vi "运维调试_总磷.vi"() -> ()   [LabVIEW 2016, in "总磷.lvlib"]
uses:
  <vilib>/Platform/TimedLoop/XDataNode/timing_clust.ctl
  <vilib>/Platform/TimedLoop/XDataNode/nitl_modes.ctl
  <vilib>/Platform/TimedLoop/XDataNode/wakeup.ctl
  <vilib>/Utility/miscctls.llb/LVPointTypeDef.ctl
  <vilib>/Platform/TimedLoop/XDataNode/XDataNode.xnode
  <vilib>/Platform/TimedLoop/XDataNode/XDNodeRunTimeDep.lvlib
panel:
  in  "数组":string[](array[string])
  in  "备用系数写入":bool
  in  "备用系数读取":bool
  in  "备用系数":T1
  in  "量程切换阈值写入":bool
  in  "量程切换阈值读取":bool
  in  "量程切换阈值":cluster{"阈值":dbl, "标液浓度":dbl}
  in  "参数下拉列表":enum16{"氨氮", "总磷"}(ring)=enum."总磷"
  in  "量程下拉列表":enum16{"低量程", "高量程"}(ring)
  in  "测量模式下拉列表":enum16{"水样测量", "空白核查", "标样核查", "盲样测试", "加标回收"}(ring)
  in  "公式":cluster{"X^2":dbl, "X":dbl, "b":dbl}
  in  "写公式":bool
  in  "读公式":bool
  in  "精度":dbl=4.0
  in  "样品5 F0":dbl
  in  "样品5 F1":dbl
  in  "样品4 F1":dbl
  in  "样品4 F0":dbl
  in  "样品3 F0":dbl
  in  "样品3 F1":dbl
  in  "样品2 F0":dbl
  in  "样品2 F1":dbl
  in  "样品1 F1":dbl
  in  "样品1 F0":dbl
  in  "method":u16(ring) items=["最小二乘", "最小绝对残差", "Bisquare"]
  in  "模型":enum32{"线性", "多项式"}(ring)
  out "r^2":dbl format="%.7g"
  out "拟合公式":string
  in  "样品2启用":bool
  in  "样品5启用":bool
  in  "样品4启用":bool
  in  "样品3启用":bool
  in  "样品1启用":bool
  in  "标液浓度5":dbl
  out "测量吸光度5":dbl
  in  "标液浓度4":dbl
  out "测量吸光度4":dbl
  in  "标液浓度3":dbl
  out "测量吸光度3":dbl
  in  "标液浓度2":dbl
  out "测量吸光度2":dbl
  out "测量吸光度1":dbl
  in  "标液浓度1":dbl
  out "XY图":cluster{"X Values":dbl[], "Y Values":dbl[]}[](graph)
  in  "返回":bool
  in  "调试":bool
  out "序列号":string="序列号"
  out "测量数据":T2(xcontrol)
  out "集成报警信息":string
  out "设置值":dbl
  out "定时启动":bool
  out "总磷总氮运行状态":T3(xcontrol)
  in  "停止":bool
  in  "手动启动":bool
  in  "单步测试":bool
  in  "总磷氨氮调试":u16[](xcontrol)
  out "F3":sgl format="%#.6f"
  out "F2":sgl format="%#.6f"
  out "F1":sgl format="%#.6f"
  out "F0":sgl format="%#.6f"
  out "多列列表框":i32(listbox)
  # "COM4"
  # "参数设置"
  # "标液浓度"
  # "F0"
  # "F1"
  # "吸光值显示"
  # "样品一"
  # "辅\n助\n计\n算\n区"
  # "样品二"
  # "样品三"
  # "样品四"
  # "样品五"
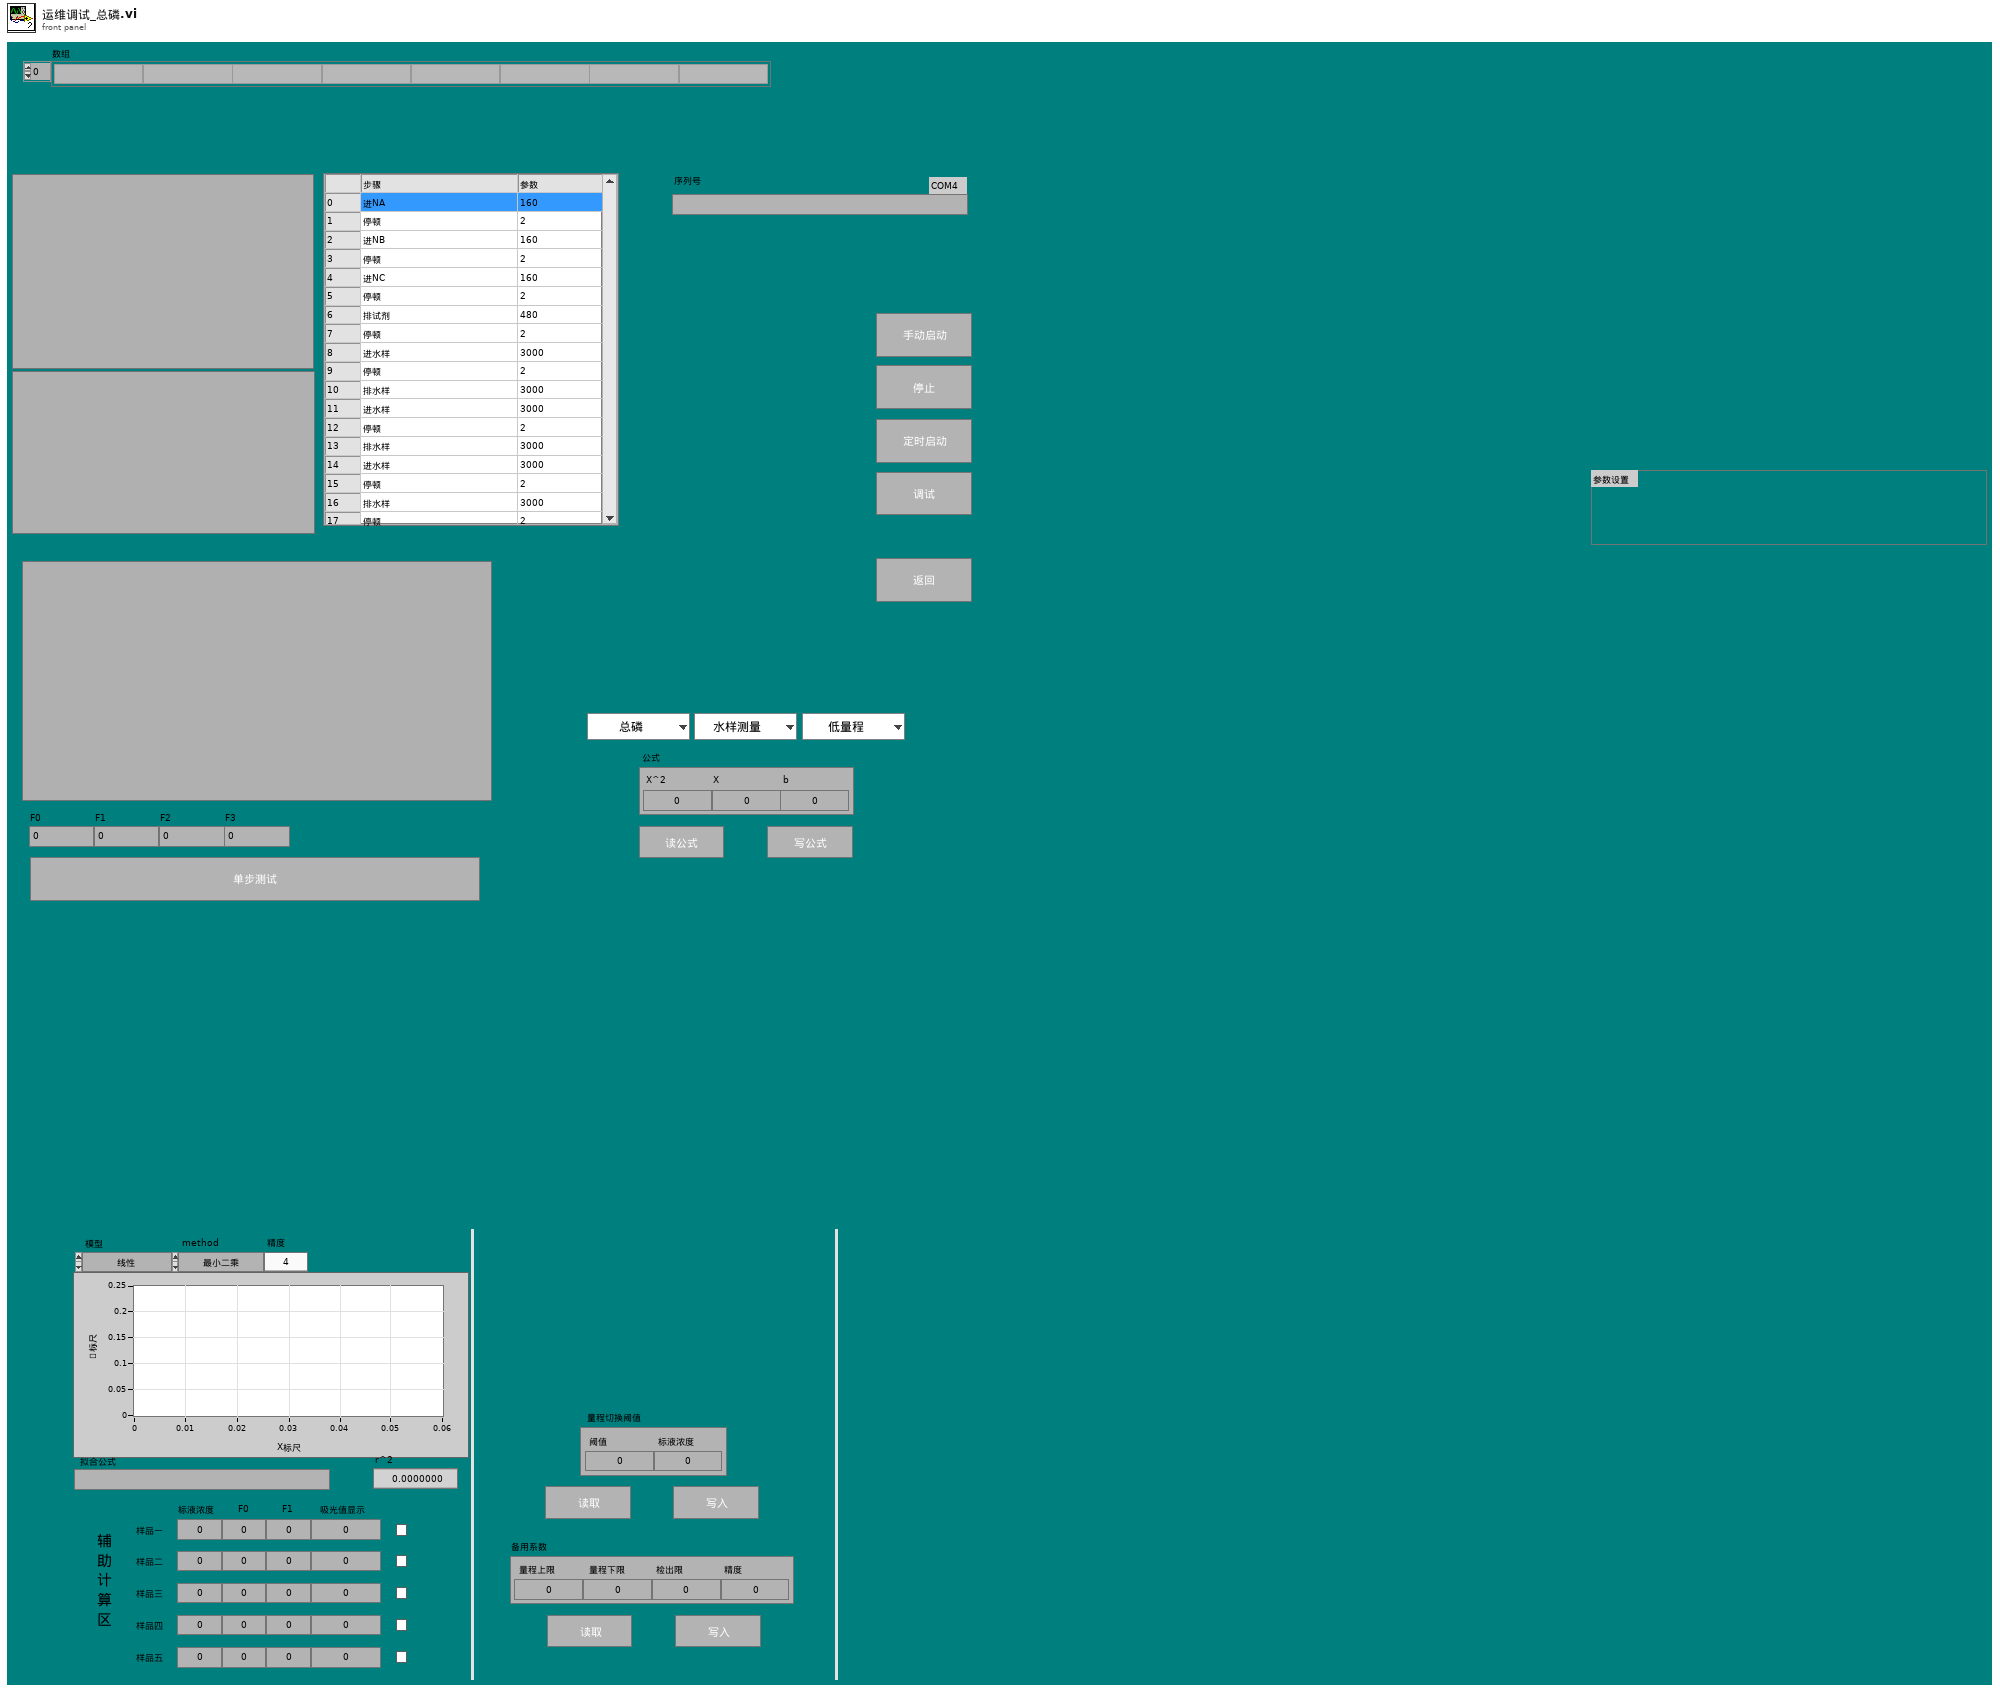
[diagram p1: front panel]
types:
  T1 = cluster{"量程上限":dbl, "量程下限":dbl, "检出限":dbl, "精度":dbl}
  T2 = cluster{"flowid":u16, "测量精度":u16, "测量数据区":cluster{"因子编码":u32, "单位":u16, "标样参考值":sgl, "水样数据时间":timestamp, "水样实测值":sgl, "水样数据标识":string, "标样数据时间":timestamp, "标样实测值":sgl, "标样数据标识":string, "空白数据时间":timestamp, "空白实测值":sgl, "空白数据标识":string, "零点核查数据时间":timestamp, "零点核查实测值":sgl, "零点核查数据标识":string, "跨度核查数据时间":timestamp, "跨度核查实测值":sgl, "跨度核查数据标识":string, "加标回收数据时间":timestamp, "加标回收实测值":sgl, "加标回收数据标识":string, "平行样数据时间":timestamp, "平行样实测值":sgl, "平行样数据标识":string}}
  T3 = cluster{"系统时间":timestamp, "工作状态":enum16{"空闲", "水样测试", "标样核查", "零点核查", "跨度核查", "空白测试", "平行样测试", "加标回收", "空白校准", "标样校准", "初始化（清洗）"}, "测量模式":enum16{"待机", "连续模式", "周期模式", "定点模式", "受控模式", "手动模式"}, "告警代码":enum16{"无告警", "缺试剂告警", "缺水样告警", "缺蒸馏水告警", "缺标液告警", "仪表漏液告警", "标定异常告警", "超量程告警", "加热异常", "低试剂预警", "超上限告警", "超下限告警", "仪表内部其他异常", "滴定异常告警", "电极异常告警", "量程切换告警", "参数设置告警", "PH电极电位异常", "电导率电极异常", "浊度光度异常", "溶解氧电极异常", "溶解氧光强异常", "温度异常告警", "PH异常告警", "溶解氧异常告警", "电导率异常告警", "浊度异常告警", "叶绿素异常告警", "藻密度异常告警", "蓝绿藻异常告警", "ORP异常告警", "氨氮异常告警", "清洁刷异常告警", "SD卡异常告警", "蓝牙异常告警", "Wifi异常告警", "流程异常告警"}, "故障代码":enum16{"无故障", "电机故障", "温度故障", "通讯故障", "滴定故障"}, "日志代码":u16, "软件版本":u16, "F0":sgl, "F1":sgl, "F2":sgl, "F3":sgl, "T":sgl, "H":sgl, "id":u16, "flowid":u16, "量程":u16}
  T4 = enum16{"待机", "启动氨氮", "氨氮测量中", "启动总磷", "总磷测量中", "延时"}
  T5 = typedef "LVPointTypeDef.ctl" = cluster{"Horizontal":i16, "Vertical":i16}
  T6 = cluster{"因子编码":u32, "单位":u16, "标样参考值":sgl, "水样数据时间":timestamp, "水样实测值":sgl, "水样数据标识":string, "标样数据时间":timestamp, "标样实测值":sgl, "标样数据标识":string, "空白数据时间":timestamp, "空白实测值":sgl, "空白数据标识":string, "零点核查数据时间":timestamp, "零点核查实测值":sgl, "零点核查数据标识":string, "跨度核查数据时间":timestamp, "跨度核查实测值":sgl, "跨度核查数据标识":string, "加标回收数据时间":timestamp, "加标回收实测值":sgl, "加标回收数据标识":string, "平行样数据时间":timestamp, "平行样实测值":sgl, "平行样数据标识":string}
  T7 = enum16{"空闲", "水样测试", "标样核查", "零点核查", "跨度核查", "空白测试", "平行样测试", "加标回收", "空白校准", "标样校准", "初始化（清洗）"}
  T8 = typedef "XDNodeRunTimeDep.lvlib/timing_clust.ctl" = cluster{"Expected End [f-1]":u64, "Actual End [f-1]":u64, "Finished Late? [f-1]":bool, "Expected End [i-1]":u64, "Actual End [i-1]":u64, "Finished Late? [i-1]":bool, "Expected Start [i]":u64, "Actual Start [i]":u64, "Expected Start [f]":u64, "Actual Start [f]":u64, "Source Name":string, "Structure Name":string, "Period":i64, "Deadline":i64, "Offset":i64, "Start":i64, "Priority":i32, "Timeout":i32, "Mode":T9, "Wakeup Reason":T10, "Error":errorcluster, "Source Type":string, "Secondary Source Type":string, "Global End Time":u64, "Global Start Time":u64, "Frame Duration":u64, "Iteration Duration":u64, "Assigned CPU":i32, "I/O Scan Engine Mode":u32}
  T9 = typedef "XDNodeRunTimeDep.lvlib/nitl_modes.ctl" = enum32{"No Change", "Process missed periods, maintain original phase", "Discard missed periods, maintain original phase", "Process missed periods, ignore original phase", "Discard missed periods, ignore original phase"}
  T10 = typedef "XDNodeRunTimeDep.lvlib/wakeup.ctl" = enum32{"Normal", "Aborted", "Asynchronous wakeup", "Timing source error", "Timed loop error", "Timeout"}
  T11 = cluster{"启动模式":enum16{"标液测量", "水样测量", "零液测量", "盲样测量", "加标回收"}, "启动参数":u16, "量程":enum16{"低量程", "高量程"}}
  T12 = cluster{"时间标识":timestamp, "设备":string, "日志信息":string, "流程参数":string}
  T13 = cluster{"时间标识":timestamp, "设备":string, "日志信息":string}
  T14 = enum16{"无告警", "缺试剂告警", "缺水样告警", "缺蒸馏水告警", "缺标液告警", "仪表漏液告警", "标定异常告警", "超量程告警", "加热异常", "低试剂预警", "超上限告警", "超下限告警", "仪表内部其他异常", "滴定异常告警", "电极异常告警", "量程切换告警", "参数设置告警", "PH电极电位异常", "电导率电极异常", "浊度光度异常", "溶解氧电极异常", "溶解氧光强异常", "温度异常告警", "PH异常告警", "溶解氧异常告警", "电导率异常告警", "浊度异常告警", "叶绿素异常告警", "藻密度异常告警", "蓝绿藻异常告警", "ORP异常告警", "氨氮异常告警", "清洁刷异常告警", "SD卡异常告警", "蓝牙异常告警", "Wifi异常告警", "流程异常告警"}
  T15 = typedef "LVRowAndColumnUnsignedTypeDef.ctl" = cluster{"Row":u32, "Column":u32}
  T16 = cluster{"站号":u16, "量程切换":enum32{"H", "L", "AUTO"}, "控制命令":enum16{"启动测量", "标样核查", "零点核查", "跨度核查", "空白测试", "平行样测试", "加标回收", "空白校准", "标样校准", "初始化（清洗）", "停止测试", "仪器重启", "校时", "模式设置", "测量间隔设置", "盲样测试"}, "模式设置":enum16{"待机", "连续模式", "周期模式", "定点模式", "受控模式", "手动模式"}, "测量间隔":u16}
  T17 = cluster{"站号":u16, "量程切换":enum32{"H", "L", "AUTO"}, "控制命令":enum16{"启动测量", "标样核查", "零点核查", "跨度核查", "空白测试", "平行样测试", "加标回收", "空白校准", "标样校准", "初始化（清洗）", "停止测试", "仪器重启", "校时", "模式设置", "测量间隔设置"}, "模式设置":enum16{"待机", "连续模式", "周期模式", "定点模式", "受控模式", "手动模式"}, "测量间隔":u16}
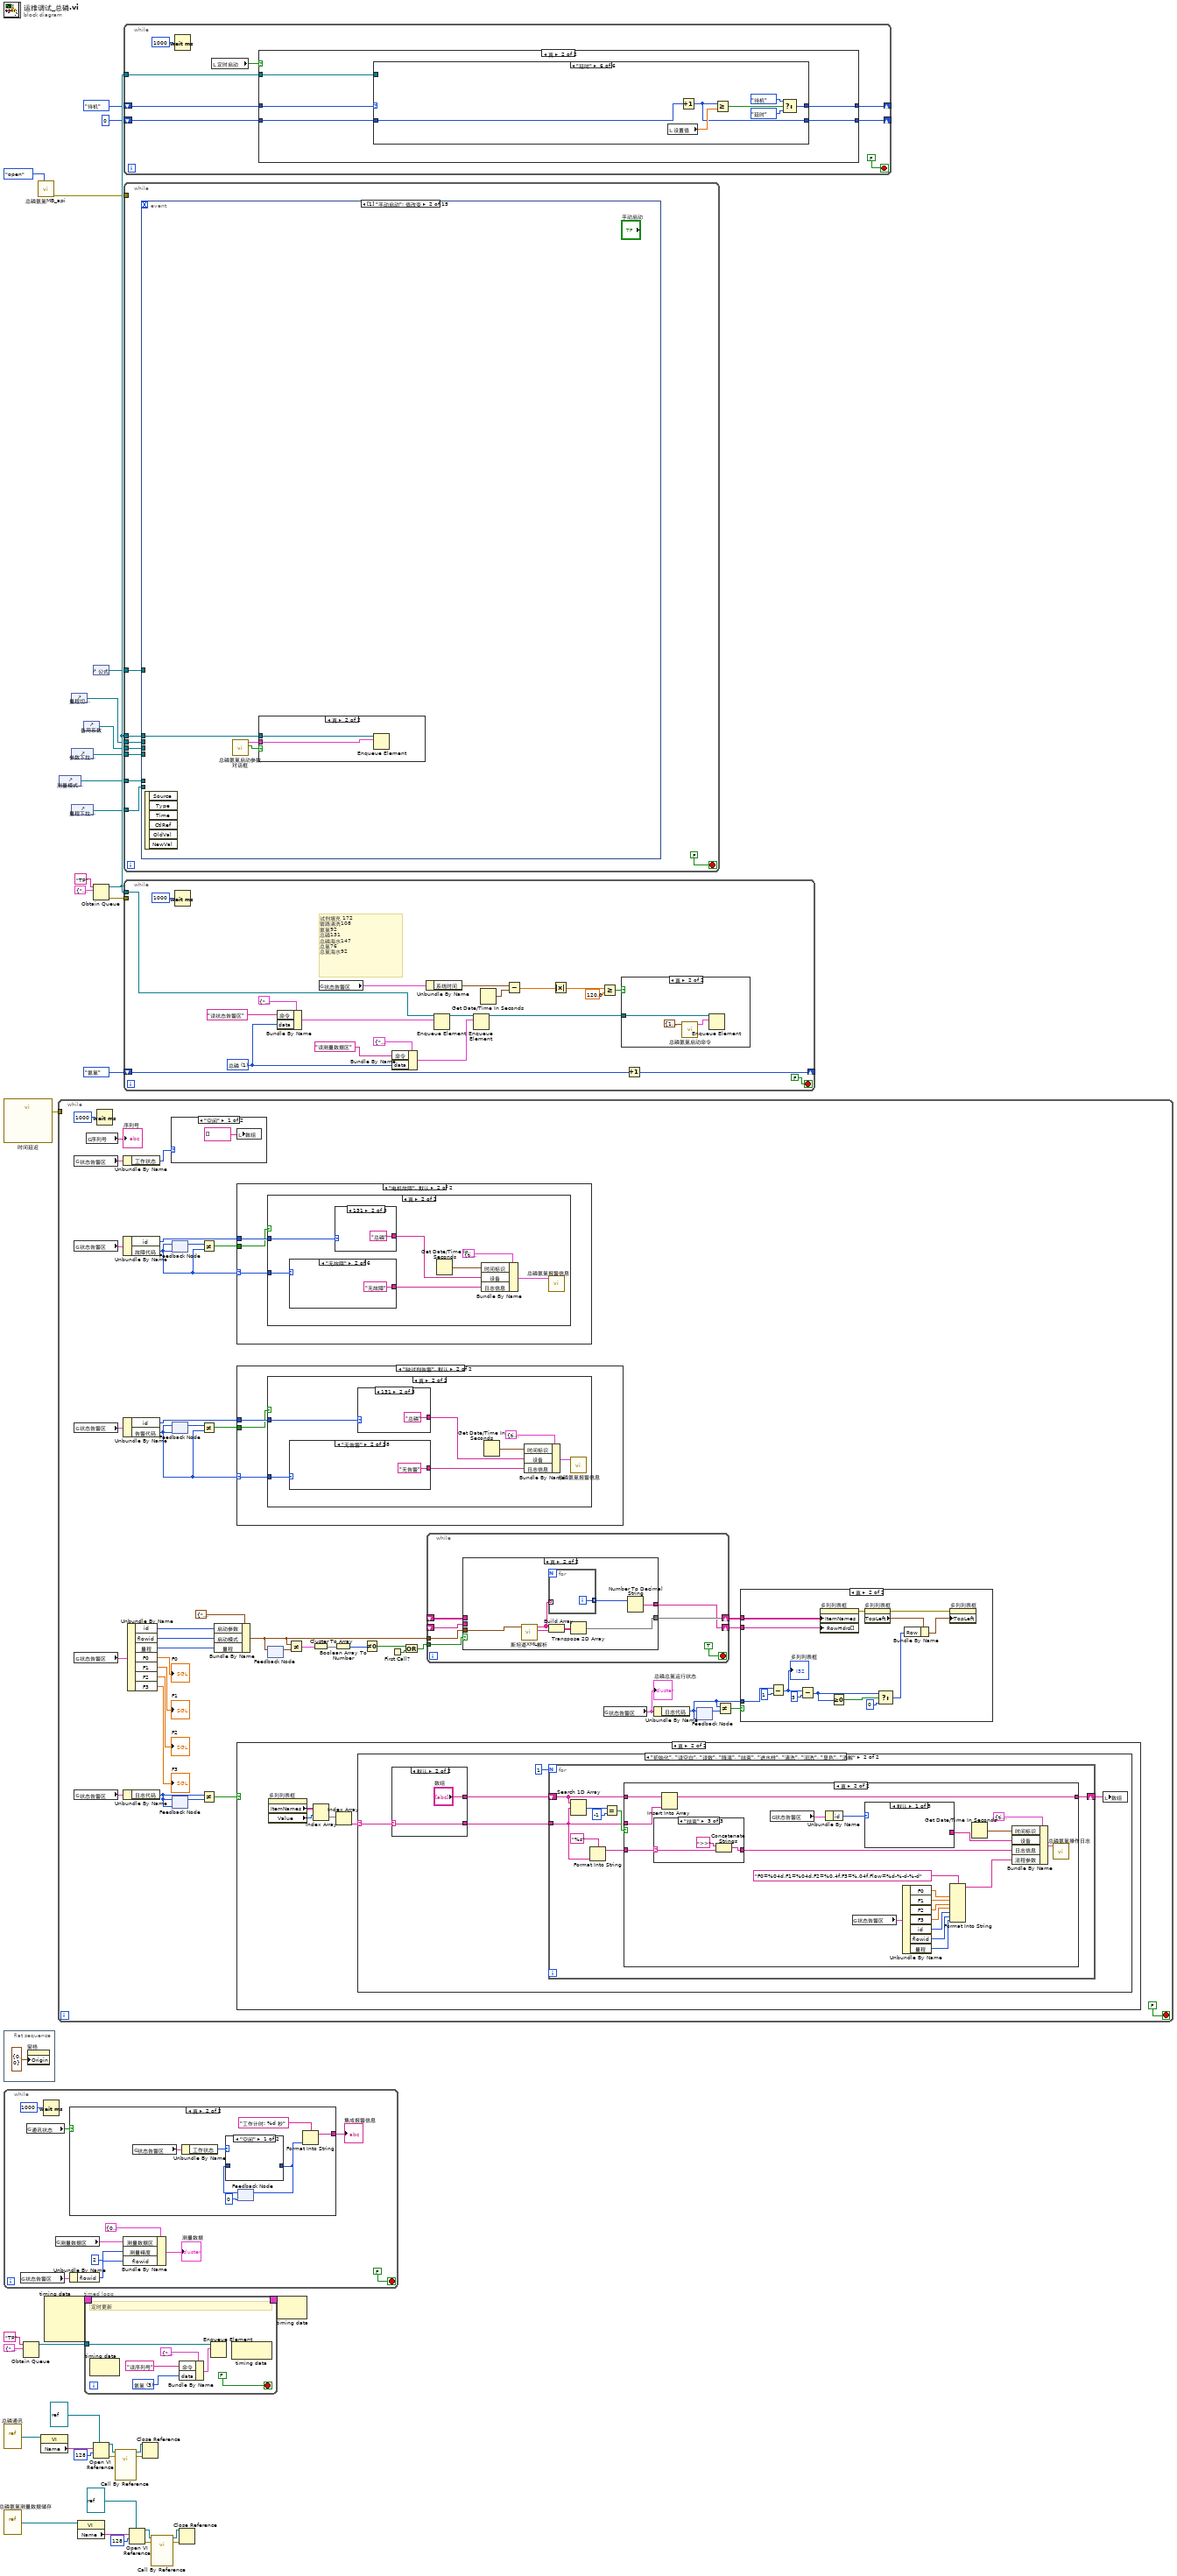
[diagram p0: block diagram]
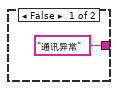
[diagram p2: hidden frame]
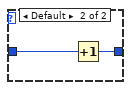
[diagram p3: hidden frame]
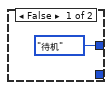
[diagram p4: hidden frame]
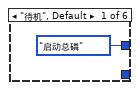
[diagram p5: hidden frame]
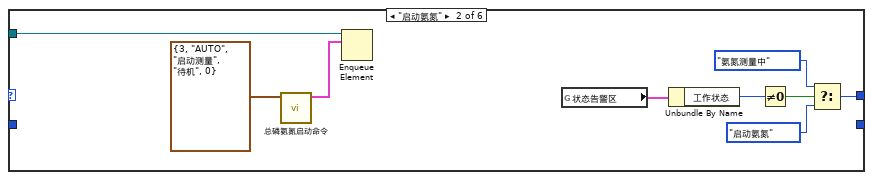
[diagram p6: hidden frame]
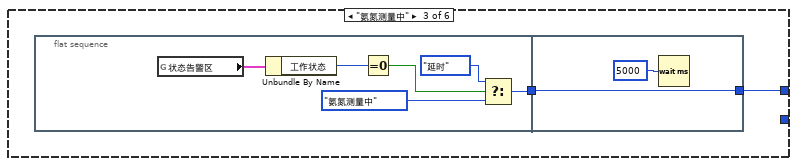
[diagram p7: hidden frame]
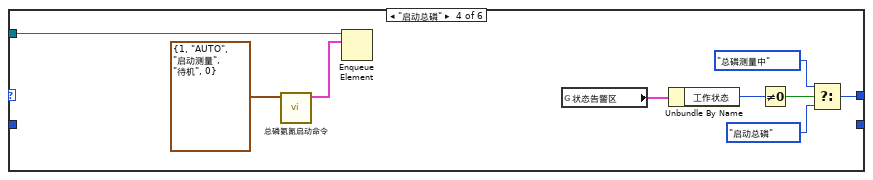
[diagram p8: hidden frame]
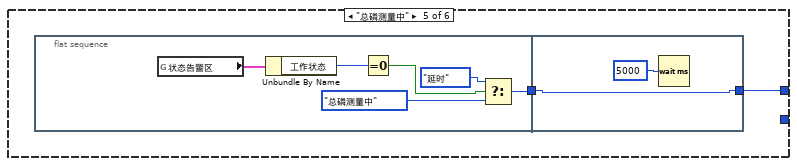
[diagram p9: hidden frame]
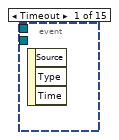
[diagram p10: hidden frame]
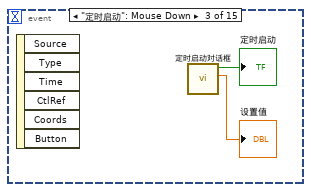
[diagram p12: hidden frame]
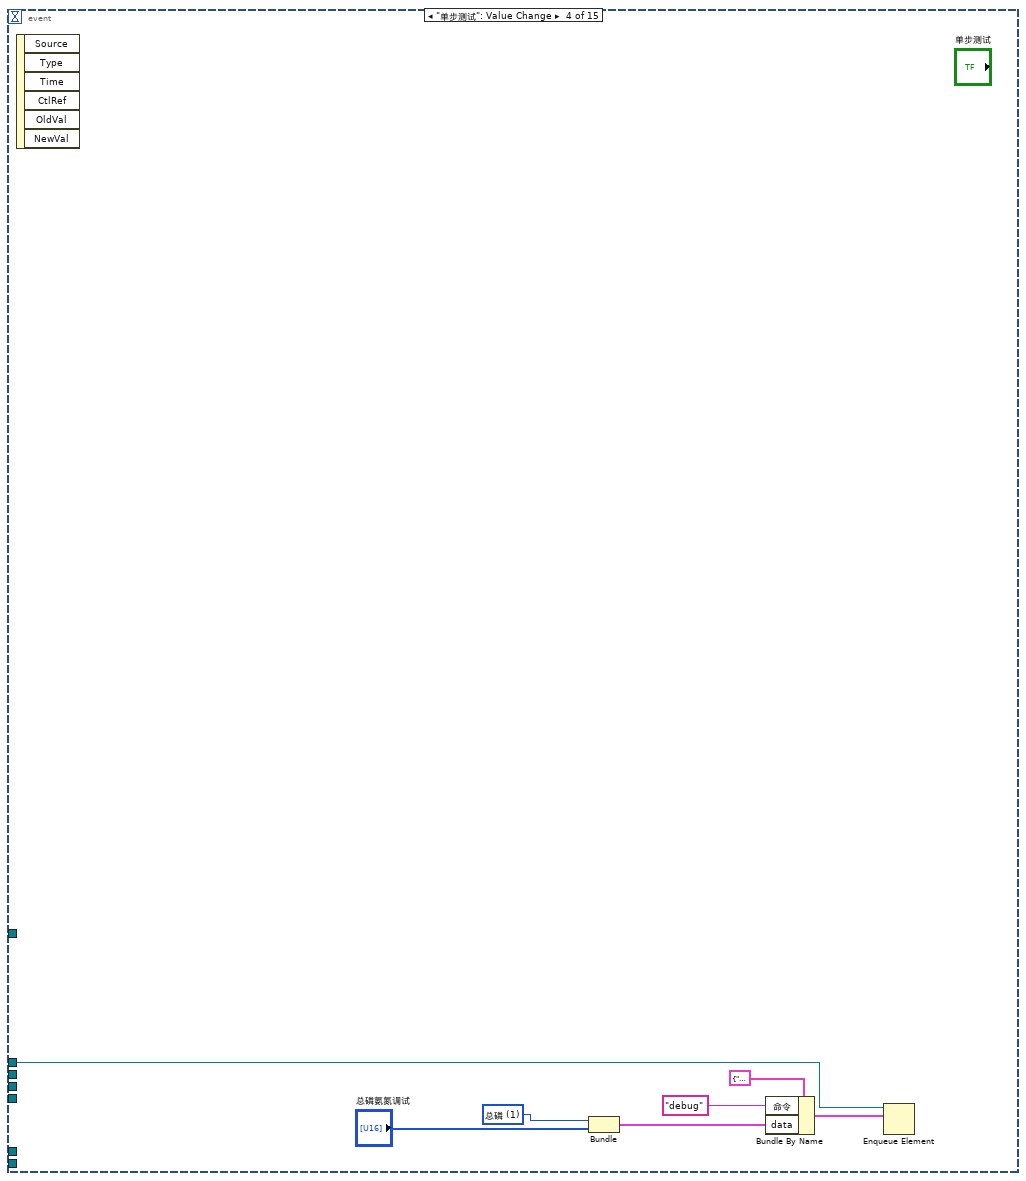
[diagram p13: hidden frame]
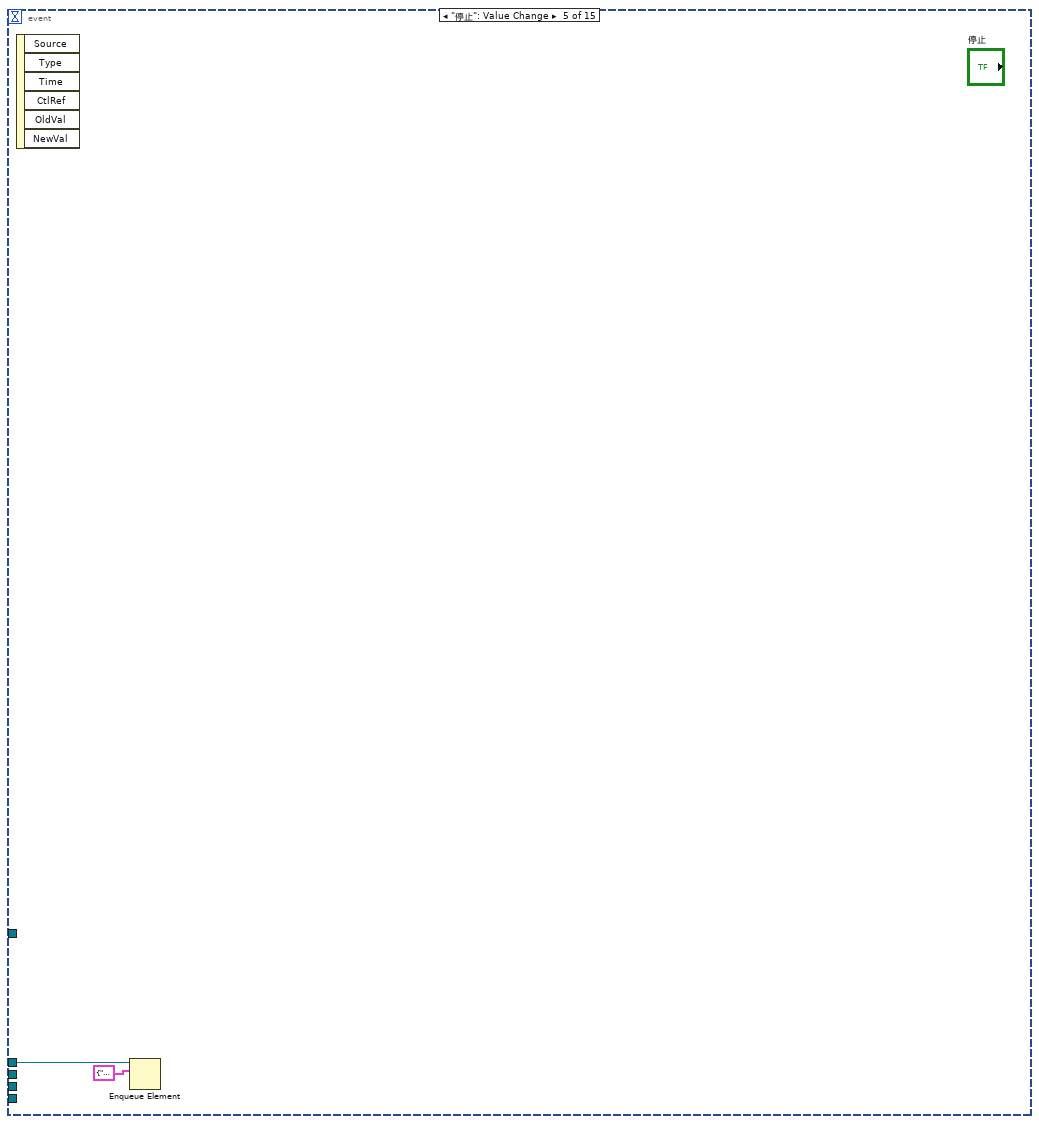
[diagram p14: hidden frame]
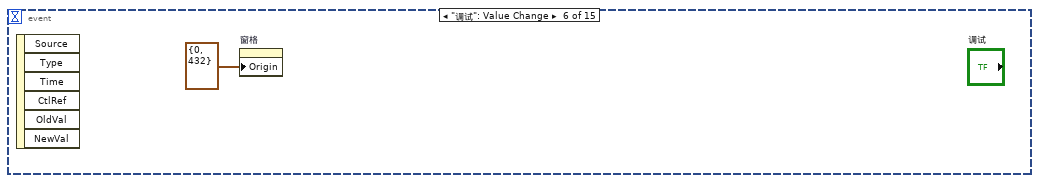
[diagram p15: hidden frame]
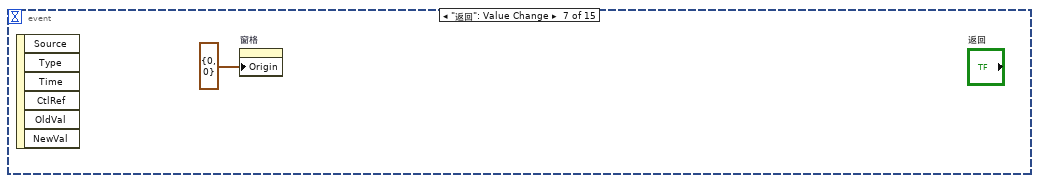
[diagram p16: hidden frame]
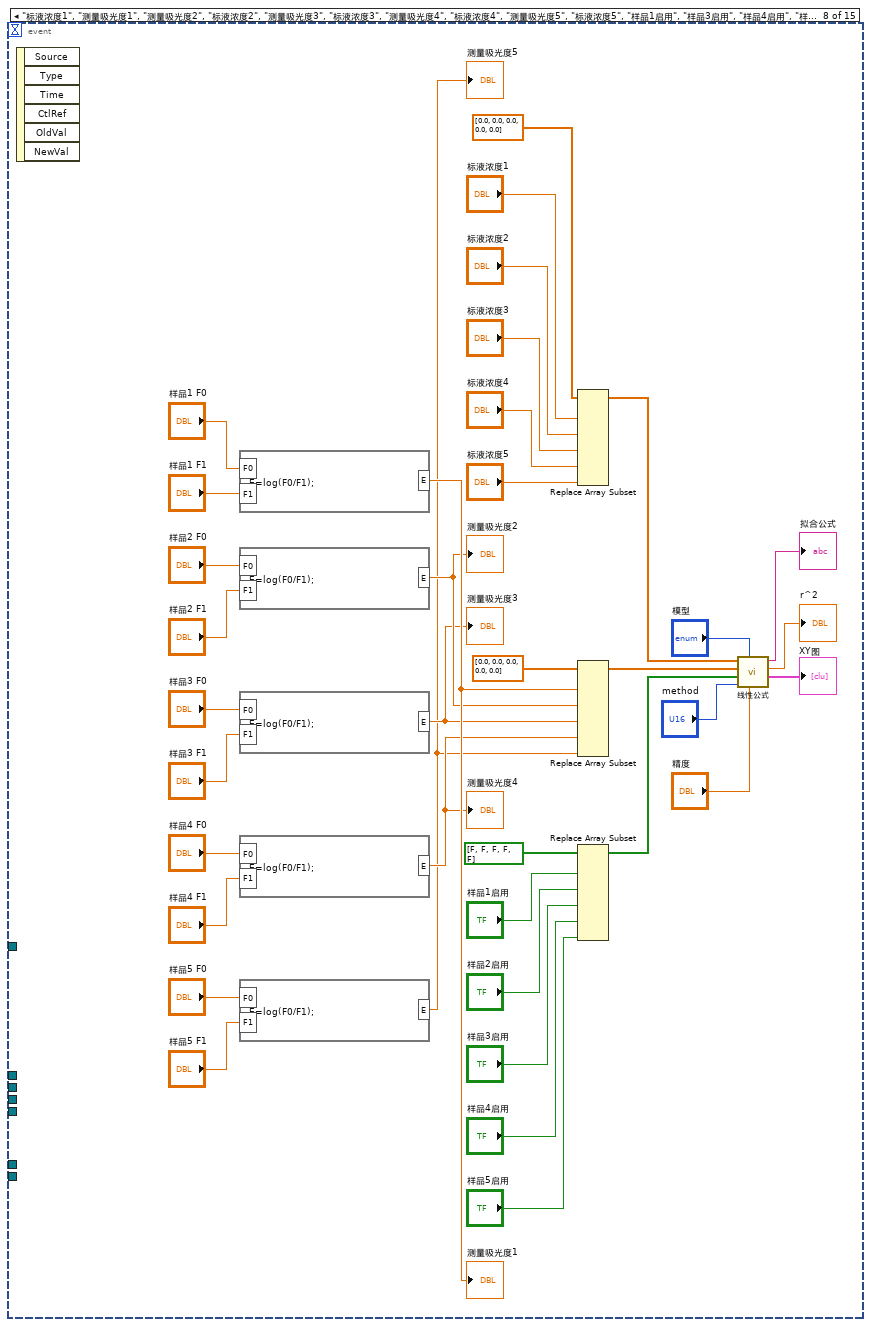
[diagram p17: hidden frame]
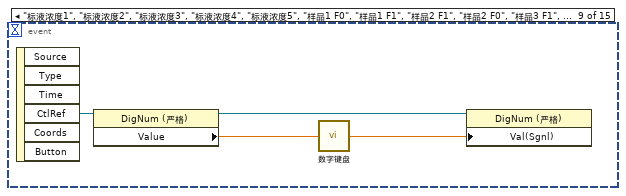
[diagram p18: hidden frame]
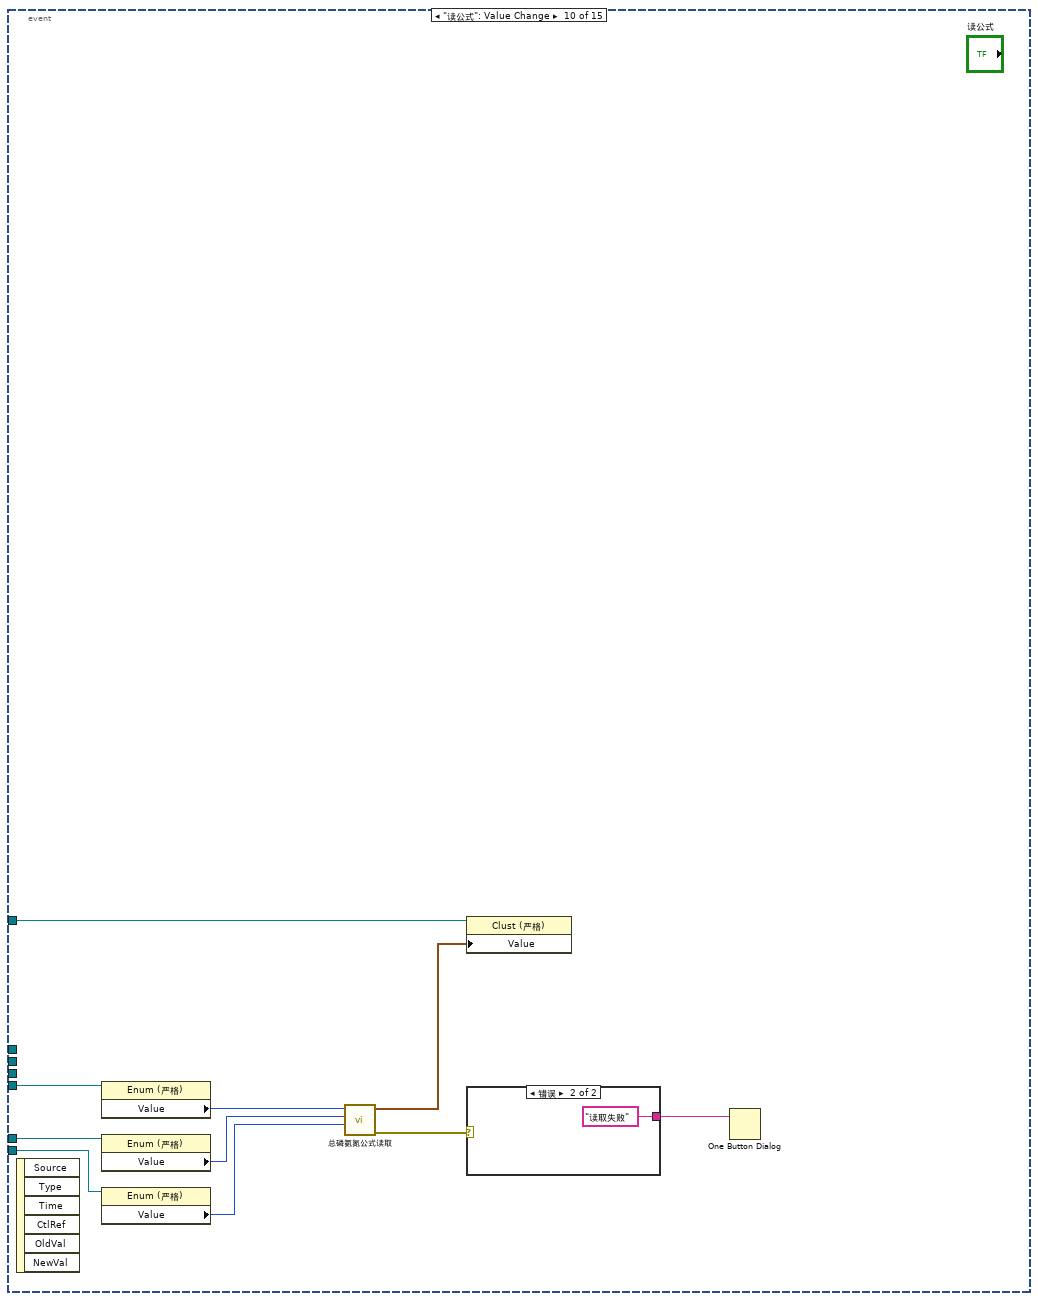
[diagram p19: hidden frame]
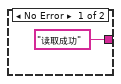
[diagram p20: hidden frame]
diagram:
  n1 = call "时间延迟"() -> ("error out"=w8:errorcluster)  [unwired: 11 in]
  n2 = flat-sequence {
    frame #0 {
      n3 = property on="窗格" class="Pane"("Origin"=T5 {"Horizontal"=0, "Vertical"=0} ("原点")) -> ()  [unwired: 2 in, 2 out]
    }
  }
  n4 = while {
    stop <- FALSE stop-if-true
    n5 = global read "VAR总磷氨氮全局变量.vi" "状态告警区"() -> (w43:T3)
    n6 = global read "VAR总磷氨氮全局变量.vi" "通讯状态"() -> (w45:bool)
    n7 = Wait (ms)(milliseconds to wait=u32 1000 ("等待时间（毫秒）")) -> ()  [unwired: 1 out]
    n8 = global read "VAR总磷氨氮全局变量.vi" "测量数据区"() -> (w46:T6)
    n9 = case shown="真" w45 {
      tunnel: ["通讯异常" ("集成报警信息") w50] -> w44
      frame False {
      }
      frame True {
        n10 = global read "VAR总磷氨氮全局变量.vi" "状态告警区"() -> (w56:T3)
        n11 = Unbundle By Name(w56) -> ("工作状态"=w55:T7)
        n12 = feedback #1(0) -> (w53:i32)
        n13 = case shown="\"空闲\"" w55 {
          tunnel: w53 -> [_ w58]
          tunnel: [_ w57] -> w51
          frame "空闲" {
          }
          frame Default {
            n14 = Increment(x=w58) -> (x+1=w57:i32)
          }
        }
        n15 = feedback-in #1(w51) -> ()
        n16 = Format Into String(format string="工作计时: %d 秒" ("格式字符串"), w51) -> (resulting string=w50:string)  [unwired: 2 in, 1 out]
      }
    }
    "集成报警信息" <- w44
    n17 = Unbundle By Name(w43) -> ("flowid"=w42:u16)
    n18 = Bundle By Name(cluster=T2 {"flowid"=0, "测量精度"=0, "测量数据区"={"因子编码"=0, "单位"=0, "标样参考值"=0.0, "水样数据时间"=timestamp(0 s since 1904-01-01), "水样实测值"=0.0, "水样数据标识"="", "标样数据时间"=timestamp(0 s since 1904-01-01), "标样实测值"=0.0, "标样数据标识"="", "空白数据时间"=timestamp(0 s since 1904-01-01), "空白实测值"=0.0, "空白数据标识"="", "零点核查数据时间"=timestamp(0 s since 1904-01-01), "零点核查实测值"=0.0, "零点核查数据标识"="", "跨度核查数据时间"=timestamp(0 s since 1904-01-01), "跨度核查实测值"=0.0, "跨度核查数据标识"="", "加标回收数据时间"=timestamp(0 s since 1904-01-01), "加标回收实测值"=0.0, "加标回收数据标识"="", "平行样数据时间"=timestamp(0 s since 1904-01-01), "平行样实测值"=0.0, "平行样数据标识"=""}} ("氨氮测量数据"), "测量数据区"=w46, "测量精度"=u16 2, "flowid"=w42) -> (→"测量数据":T2)
  }
  n19 = vi-ref "总磷通讯.vi"() -> (w31:refnum<vi>)
  n20 = vi-ref "总磷氨氮测量数据储存.vi"() -> (w23:refnum<vi>)
  n21 = Obtain Queue(name (unnamed)="TP" ("名称（未命名）"), element data type=cluster{"命令":string, "data":variant} {"命令"="", "data"=variant}) -> (queue out=w1:refnum<queue>)  [unwired: 3 in, 2 out]
  n22 = call "总磷氨氮MB_api.vi"("STEP"=enum16{"open", "read", "write", "close"}."open") -> ("error out"=w7:errorcluster)  [unwired: 8 in, 2 out]
  n23 = property class="VI"(reference=w31) -> ("Name"=w30:string)  [unwired: 1 in, 2 out]
  n24 = node-c288() -> (w5:T8)  [unwired: 4 in]
  n25 = while {
    tunnel: w8 -> [_]
    stop <- FALSE stop-if-true
    n26 = global read "VAR总磷氨氮全局变量.vi" "状态告警区"() -> (w64:T3)
    n27 = global read "VAR总磷氨氮全局变量.vi" "状态告警区"() -> (w70:T3)
    n28 = global read "VAR总磷氨氮全局变量.vi" "状态告警区"() -> (w75:T3)
    n29 = global read "VAR总磷氨氮全局变量.vi" "状态告警区"() -> (w87:T3)
    n30 = global read "VAR总磷氨氮全局变量.vi" "状态告警区"() -> (w61:T3)
    n31 = global read "VAR总磷氨氮全局变量.vi" "序列号"() -> (→"序列号":string)
    n32 = Wait (ms)(milliseconds to wait=u32 1000 ("等待时间（毫秒）")) -> ()  [unwired: 1 out]
    n33 = Unbundle By Name(w64) -> ("工作状态"=w63:T7)
    n34 = Unbundle By Name(w70) -> ("id"=w69:u16, "故障代码"=w66:enum16{"无故障", "电机故障", "温度故障", "通讯故障", "滴定故障"})
    n35 = Unbundle By Name(w75) -> ("id"=w74:u16, "告警代码"=w71:T14)
    n36 = Unbundle By Name(w61) -> ("日志代码"=w60:u16)
    n37 = Unbundle By Name(w87) -> ("id"=w84:u16, "flowid"=w86:u16, "量程"=w85:u16, "F0"=→"F0":sgl, "F1"=→"F1":sgl, "F2"=→"F2":sgl, "F3"=→"F3":sgl)
    n38 = case shown="\"空闲\"" w63 {
      frame "空闲" {
        n39 = local write "数组"(string[] [] ("数组")) -> ()
      }
      frame "水样测试", Default {
      }
    }
    n40 = feedback #2(w66) -> (w67:enum16{"无故障", "电机故障", "温度故障", "通讯故障", "滴定故障"})
    n41 = feedback-in #2(w66) -> ()
    n42 = feedback #3(w71) -> (w72:T14)
    n43 = feedback-in #3(w71) -> ()
    n44 = feedback #4(w60) -> (w62:u16)
    n45 = feedback-in #4(w60) -> ()
    n46 = Not Equal?(x=w67, y=w66) -> (x != y?=w68:bool)
    n47 = Not Equal?(x=w72, y=w71) -> (x != y?=w73:bool)
    n48 = Not Equal?(x=w60, y=w62) -> (x != y?=w59:bool)
    n49 = Bundle By Name(cluster=T11 {"启动模式"=enum."加标回收", "启动参数"=1, "量程"=enum."低量程"} ("参数簇"), "启动参数"=w84, "启动模式"=w86, "量程"=w85) -> (w77:T11)
    n50 = case shown="\"电机故障\", 默认" w66 {
      selector: w66 -> [_ w155]
      tunnel: w69 -> [_ w156]
      tunnel: w68 -> [_ w154]
      frame "无故障" {
      }
      frame "电机故障", Default {
        n51 = case shown="真" w154 {
          tunnel: w156 -> [_ w163]
          tunnel: w155 -> [_ w158]
          frame False {
          }
          frame True {
            n52 = case shown="\"无故障\"" w158 {
              selector: w158 -> [w165 _ _ _ _ _]
              tunnel: [w164 "无故障" "电机故障" "温度故障" "通讯故障" "滴定故障"] -> w157
              frame Default {
                n53 = Format Into String(format string="%d" ("格式字符串"), initial string="未知" ("工作状态"), w165) -> (resulting string=w164:string)  [unwired: 1 in, 1 out]
              }
              frame "无故障" {
              }
              frame "电机故障" {
              }
              frame "温度故障" {
              }
              frame "通讯故障" {
              }
              frame "滴定故障" {
              }
            }
            n54 = case shown="131" w163 {
              tunnel: [_ "总磷" ("table输入") "氨氮" ("table输入")] -> w159
              frame Default {
              }
              frame 131 {
              }
              frame 92 {
              }
            }
            n55 = Get Date/Time In Seconds() -> (seconds since 1Jan1904=w160:timestamp)
            n56 = Bundle By Name(cluster=T13 {"时间标识"=timestamp(0 s since 1904-01-01), "设备"="", "日志信息"=""} ("data in"), "时间标识"=w160, "设备"=w159, "日志信息"=w157) -> (w161:T13)
            n57 = call "总磷氨氮报警信息.vi"("data in"=w161) -> ()  [unwired: 11 in]
          }
        }
      }
    }
    n58 = case shown="\"缺试剂告警\", 默认" w71 {
      selector: w71 -> [_ w176]
      tunnel: w74 -> [_ w177]
      tunnel: w73 -> [_ w175]
      frame "无告警" {
      }
      frame "缺试剂告警", Default {
        n59 = case shown="真" w175 {
          tunnel: w177 -> [_ w184]
          tunnel: w176 -> [_ w178]
          frame False {
          }
          frame True {
            n60 = case shown="\"无告警\"" w178 {
              selector: w178 -> [w186 _ _ _ _ _ _ _ _ _ _ _ _ _ _ _ _ _ _ _ _ _ _ _ _ _ _ _ _ _ _ _ _ _ _ _ _ _]
              tunnel: [w185 "无告警" "缺试剂告警" "缺水样告警" "缺蒸馏水告警" "缺标液告警" "仪表漏液告警" "标定异常告警" "超量程告警" "加热异常" "低试剂预警" "超上限告警" "超下限告警" "仪表内部其他异常" "滴定异常告警" "电极异常告警" "量程切换告警" "参数设置告警" "PH电极电位异常" "电导率电极异常" "浊度光度异常" "溶解氧电极异常" "溶解氧光强异常" "温度异常告警" "PH异常告警" "溶解氧异常告警" "电导率异常告警" "浊度异常告警" "叶绿素异常告警" "藻密度异常告警" "蓝绿藻异常告警" "ORP异常告警" "氨氮异常告警" "清洁刷异常告警" "SD卡异常告警" "蓝牙异常告警" "WiFi异常告警" "流程异常告警"] -> w179
              frame Default {
                n61 = Format Into String(format string="%d" ("格式字符串"), initial string="未知" ("工作状态"), w186) -> (resulting string=w185:string)  [unwired: 1 in, 1 out]
              }
              frame "无告警" {
              }
              frame "缺试剂告警" {
              }
              frame "缺水样告警" {
              }
              frame "缺蒸馏水告警" {
              }
              frame "缺标液告警" {
              }
              frame "仪表漏液告警" {
              }
              frame "标定异常告警" {
              }
              frame "超量程告警" {
              }
              frame "加热异常" {
              }
              frame "低试剂预警" {
              }
              frame "超上限告警" {
              }
              frame "超下限告警" {
              }
              frame "仪表内部其他异常" {
              }
              frame "滴定异常告警" {
              }
              frame "电极异常告警" {
              }
              frame "量程切换告警" {
              }
              frame "参数设置告警" {
              }
              frame "PH电极电位异常" {
              }
              frame "电导率电极异常" {
              }
              frame "浊度光度异常" {
              }
              frame "溶解氧电极异常" {
              }
              frame "溶解氧光强异常" {
              }
              frame "温度异常告警" {
              }
              frame "PH异常告警" {
              }
              frame "溶解氧异常告警" {
              }
              frame "电导率异常告警" {
              }
              frame "浊度异常告警" {
              }
              frame "叶绿素异常告警" {
              }
              frame "藻密度异常告警" {
              }
              frame "蓝绿藻异常告警" {
              }
              frame "ORP异常告警" {
              }
              frame "氨氮异常告警" {
              }
              frame "清洁刷异常告警" {
              }
              frame "SD卡异常告警" {
              }
              frame "蓝牙异常告警" {
              }
              frame "Wifi异常告警" {
              }
              frame "流程异常告警" {
              }
            }
            n62 = case shown="131" w184 {
              tunnel: [_ "总磷" ("table输入") "氨氮" ("table输入")] -> w180
              frame Default {
              }
              frame 131 {
              }
              frame 92 {
              }
            }
            n63 = Get Date/Time In Seconds() -> (seconds since 1Jan1904=w181:timestamp)
            n64 = Bundle By Name(cluster=T13 {"时间标识"=timestamp(0 s since 1904-01-01), "设备"="", "日志信息"=""} ("data in"), "时间标识"=w181, "设备"=w180, "日志信息"=w179) -> (w182:T13)
            n65 = call "总磷氨氮报警信息.vi"("data in"=w182) -> ()  [unwired: 11 in]
          }
        }
      }
    }
    n66 = case shown="真" w59 {
      frame False {
      }
      frame True {
        n67 = property on="多列列表框" class="MCListbox (严格)"() -> ("ItemNames"=w104:string[][], "Value"=w105:i32)  [unwired: 2 in, 2 out]
        n68 = Index Array(array=w104, index (row)=w105) -> (element=w103:string[])  [unwired: 1 in]
        n69 = Index Array(array=w103) -> (element=w102:string)  [unwired: 1 in]
        n70 = case shown="\"初始化\", \"读空白\", \"读数\", \"降温\", \"结束\", \"进水样\", \"清洗\", \"润洗\", \"显色\", \"消解\"" w102 {
          selector: w102 -> [_ w108]
          frame Default {
          }
          frame "初始化", "读空白", "读数", "降温", "结束", "进水样", "清洗", "润洗", "显色", "消解" {
            n71 = case shown="默认" w108 {
              selector: w108 -> [w112 w114]
              tunnel: [w112 w114] -> w107
              tunnel: [string[] [] ("数组") "数组"] -> w106
              frame "读数" {
              }
              frame Default {
              }
            }
            n72 = for {
              N: 1 -> [_]
              tunnel: w107 -> [w116]
              shift-right: [w115] -> w109
              shift-left: w106 -> [w117]
              n73 = Search 1D Array(1D array=w117, element=w116) -> (index of element=w120:i32)  [unwired: 1 in]
              n74 = Format Into String(format string="%s" ("格式字符串"), w116) -> (resulting string=w121:string)  [unwired: 2 in, 1 out]
              n75 = Equal?(x=w120, y=-1) -> (x = y?=w118:bool)
              n76 = case shown="真" w118 {
                tunnel: w121 -> [_ w125]
                tunnel: w117 -> [w123 w129]
                tunnel: w116 -> [_ w128]
                tunnel: [w123 w127] -> w115
                frame False {
                }
                frame True {
                  n77 = case shown="\"结束\"" w125 {
                    selector: w125 -> [w145 w148 w151]
                    tunnel: [w145 w147 w150] -> w124
                    frame Default {
                    }
                    frame "初始化" {
                      n78 = Concatenate Strings("<<" ("字符串"), w148) -> (w147:string)
                    }
                    frame "结束" {
                      n79 = Concatenate Strings(">>" ("字符串"), w151) -> (w150:string)
                    }
                  }
                  n80 = Insert Into Array(array=w129, new element=w128) -> (w127:string[])  [unwired: 1 in]
                  n81 = global read "VAR总磷氨氮全局变量.vi" "状态告警区"() -> (w144:T3)
                  n82 = Unbundle By Name(w144) -> ("id"=w143:u16)
                  n83 = global read "VAR总磷氨氮全局变量.vi" "状态告警区"() -> (w139:T3)
                  n84 = case shown="默认" w143 {
                    tunnel: [_ "总磷" ("table输入") "氨氮" ("table输入")] -> w141
                    frame Default {
                    }
                    frame 131 {
                    }
                    frame 92 {
                    }
                  }
                  n85 = Unbundle By Name(w139) -> ("F0"=w136:sgl, "F1"=w135:sgl, "F2"=w134:sgl, "F3"=w133:sgl, "id"=w132:u16, "flowid"=w131:u16, "量程"=w130:u16)
                  n86 = Format Into String(format string="F0=%04d,F1=%04d,F2=%0.4f,F3=%.04f,Flow=%d-%-d-%-d" ("格式字符串"), w136, w135, w134, w133, w132, w131, w130) -> (resulting string=w137:string)  [unwired: 2 in, 1 out]
                  n87 = Get Date/Time In Seconds() -> (seconds since 1Jan1904=w140:timestamp)
                  n88 = Bundle By Name(cluster=T12 {"时间标识"=timestamp(0 s since 1904-01-01), "设备"="", "日志信息"="", "流程参数"=""} ("data in"), "时间标识"=w140, "设备"=w141, "日志信息"=w124, "流程参数"=w137) -> (w142:T12)
                  n89 = call "总磷氨氮操作日志.vi"("data in"=w142) -> ()  [unwired: 11 in]
                }
              }
            }
            n90 = local write "数组"(w109) -> ()
          }
        }
      }
    }
    n91 = feedback #5() -> (w93:T11)  [unwired: 1 in]
    n92 = feedback-in #5(w77) -> ()
    n93 = Not Equal?(x=w77, y=w93) -> (x != y?=w94:cluster{"启动模式":bool, "启动参数":bool, "量程":bool})
    n94 = Cluster To Array(cluster=w94) -> (array=w95:bool[])
    n95 = Boolean Array To Number(Boolean array=w95) -> (number=w96:u32)
    n96 = Not Equal To 0?(x=w96) -> (x != 0?=w89:bool)
    n97 = First Call?() -> (First Call?: T/F=w90:bool)
    n98 = Or(x=w89, y=w90) -> (x .or. y?=w88:bool)
    n99 = while {
      tunnel: w88 -> [w234]
      tunnel: w77 -> [w233]
      shift-right: [w232] -> w92
      shift-left: _ -> [w228]
      shift-right: [w231] -> w91
      shift-left: _ -> [w229]
      stop <- TRUE stop-if-true
      n100 = case shown="真" w234 {
        tunnel: [w236 w243] -> w231
        tunnel: [w235 w242] -> w232
        tunnel: w233 -> [_ w237]
        tunnel: w229 -> [w236 _]
        tunnel: w228 -> [w235 _]
        frame False {
        }
        frame True {
          n101 = call "斯坦道XML解析.vi"("参数簇"=w237) -> ("步骤时间"=w238:string[], "步骤名"=w240:string[])  [unwired: 9 in]
          n102 = for {
            tunnel: w240 -> [_] mode=indexing
            tunnel: [w244] -> w241 mode=indexing
            i -> [w244]
          }
          n103 = Build Array(w240, w238) -> (w239:string[][])
          n104 = Transpose 2D Array(2D array=w239) -> (transposed array=w242:string[][])
          n105 = Number To Decimal String(number=w241) -> (decimal integer string=w243:string[])  [unwired: 1 in]
        }
      }
    }
    n106 = global read "VAR总磷氨氮全局变量.vi" "状态告警区"() -> (w78:T3)
    "总磷总氮运行状态" <- w78
    n107 = Unbundle By Name(w78) -> ("日志代码"=w65:u16)
    n108 = feedback-in #6(w65) -> ()
    n109 = feedback #6(w65) -> (w98:u16)
    n110 = Not Equal?(x=w65, y=w98) -> (x != y?=w97:bool)
    n111 = case shown="真" w97 {
      tunnel: w65 -> [_ w247]
      tunnel: w92 -> [_ w254]
      tunnel: w91 -> [_ w253]
      frame False {
      }
      frame True {
        n112 = Subtract(x=w247, y=1) -> (x-y=w245:i32)
        "多列列表框" <- w245
        n113 = Subtract(x=w245, y=5) -> (x-y=w249:i32)
        n114 = property on="多列列表框" class="MCListbox (严格)"("ItemNames"=w254, "RowHdrs[]"=w253) -> (error out=w255:errorcluster)  [unwired: 2 in, 1 out]
        n115 = Greater Or Equal To 0?(x=w249) -> (x >= 0?=w248:bool)
        n116 = property on="多列列表框" class="MCListbox (严格)"(error in=w255) -> (error out=w256:errorcluster, "TopLeft"=w257:T15)  [unwired: 1 in, 1 out]
        n117 = Select(t=w249, s=w248, f=0) -> (s? t:f=w250:i32)
        n118 = Bundle By Name(cluster=w257, "Row"=w250) -> (w258:T15)
        n119 = property on="多列列表框" class="MCListbox (严格)"(error in=w256, "TopLeft"=w258) -> ()  [unwired: 1 in, 2 out]
      }
    }
  }
  n120 = control-ref of="测量模式下拉列表"() -> (w12:refnum<vi>)
  n121 = control-ref of="量程切换阈值"() -> (w10:refnum<vi>)
  n122 = control-ref of="参数下拉列表"() -> (w13:refnum<vi>)
  n123 = control-ref of="量程下拉列表"() -> (w14:refnum<vi>)
  n124 = property class="VI"(reference=w23) -> ("Name"=w16:string)  [unwired: 1 in, 2 out]
  n125 = control-ref of="备用系数"() -> (w9:refnum<vi>)
  n126 = timed-loop {
    timing: w5 -> [_]
    timing-out: [_] -> w4
    tunnel: w1 -> [w260]
    stop <- FALSE stop-if-true
    w261 = u16 3 items=["总磷"=1, "氨氮"=3] ("站号")
    # "定时更新"
    n127 = node-c288() -> ()  [unwired: 1 in, 1 out]
    n128 = Bundle By Name(cluster=cluster{"命令":string, "data":variant} {"命令"="", "data"=variant} ("元素"), "命令"="读序列号", "data"=w261) -> (w259:cluster{"命令":string, "data":variant})
    n129 = Enqueue Element(queue=w260, element=w259) -> ()  [unwired: 2 in, 3 out]
    n130 = node-c288() -> ()  [unwired: 1 in, 1 out]
  }
  n131 = control-ref of="公式"() -> (w11:refnum<vi>)
  n132 = Open VI Reference(type specifier VI Refnum (for type only)=refnum<vi> refnum, vi path=w30, options=128 ("选项")) -> (vi reference=w28:refnum<vi>, error out=w26:errorcluster)  [unwired: 3 in]
  n133 = Obtain Queue(name (unnamed)="TP" ("名称（未命名）"), element data type=cluster{"命令":string, "data":variant} {"命令"="", "data"=variant}) -> (queue out=w34:refnum<queue>, error out=w35:errorcluster)  [unwired: 3 in, 1 out]
  n134 = call-by-ref "?"(reference=w28, error in=w26) -> (reference out=w24:refnum<vi>, error out=w25:errorcluster)  [unwired: 12 in]
  n135 = while {
    tunnel: w34 -> [w269]
    shift-right: [w270] -> _
    shift-left: T4."待机" -> [w271]
    shift-right: [w267] -> _
    shift-left: u32 0 ("等待时间（毫秒）") -> [w268]
    stop <- FALSE stop-if-true
    n136 = Wait (ms)(milliseconds to wait=u32 1000 ("等待时间（毫秒）")) -> ()  [unwired: 1 out]
    n137 = local read "定时启动"() -> (w272:bool)
    n138 = case shown="真" w272 {
      tunnel: w271 -> [_ w280]
      tunnel: [T4."待机" w279] -> w270
      tunnel: w269 -> [_ w278]
      tunnel: w268 -> [_ w277]
      tunnel: [_ w276] -> w267
      frame False {
      }
      frame True {
        n139 = case shown="\"延时\"" w280 {
          tunnel: [T4."启动总磷" w285 w292 w303 w311 w323] -> w279
          tunnel: w278 -> [_ w290 _ w309 _ _]
          tunnel: w277 -> [_ _ _ _ _ w326]
          tunnel: [_ _ _ _ _ w322] -> w276
          frame "待机", Default {
          }
          frame "启动氨氮" {
            n140 = call "总磷氨氮启动命令.vi"("参数"=T16 {"站号"=3, "量程切换"=enum."AUTO", "控制命令"=enum."启动测量", "模式设置"=enum."待机", "测量间隔"=0}) -> ("启动命令"=w283:cluster{"命令":string, "data":variant})  [unwired: 10 in]
            n141 = Enqueue Element(queue=w290, element=w283) -> ()  [unwired: 2 in, 3 out]
            n142 = global read "VAR总磷氨氮全局变量.vi" "状态告警区"() -> (w289:T3)
            n143 = Unbundle By Name(w289) -> ("工作状态"=w288:T7)
            n144 = Not Equal To 0?(x=w288) -> (x != 0?=w287:bool)
            n145 = Select(t=T4."氨氮测量中", s=w287, f=T4."启动氨氮") -> (s? t:f=w285:T4)
          }
          frame "氨氮测量中" {
            n146 = flat-sequence {
              tunnel: [w296] -> w291
              tunnel: [w300] -> w292
              tunnel: w291 -> [w300]
              frame #0 {
                n147 = global read "VAR总磷氨氮全局变量.vi" "状态告警区"() -> (w297:T3)
                n148 = Unbundle By Name(w297) -> ("工作状态"=w298:T7)
                n149 = Equal To 0?(x=w298) -> (x = 0?=w293:bool)
                n150 = Select(t=T4."延时", s=w293, f=T4."氨氮测量中") -> (s? t:f=w296:T4)
              }
              frame #1 {
                n151 = Wait (ms)(milliseconds to wait=u32 5000 ("等待时间（毫秒）")) -> ()  [unwired: 1 out]
              }
            }
          }
          frame "启动总磷" {
            n152 = call "总磷氨氮启动命令.vi"("参数"=T16 {"站号"=1, "量程切换"=enum."AUTO", "控制命令"=enum."启动测量", "模式设置"=enum."待机", "测量间隔"=0}) -> ("启动命令"=w302:cluster{"命令":string, "data":variant})  [unwired: 10 in]
            n153 = Enqueue Element(queue=w309, element=w302) -> ()  [unwired: 2 in, 3 out]
            n154 = global read "VAR总磷氨氮全局变量.vi" "状态告警区"() -> (w304:T3)
            n155 = Unbundle By Name(w304) -> ("工作状态"=w305:T7)
            n156 = Not Equal To 0?(x=w305) -> (x != 0?=w306:bool)
            n157 = Select(t=T4."总磷测量中", s=w306, f=T4."启动总磷") -> (s? t:f=w303:T4)
          }
          frame "总磷测量中" {
            n158 = flat-sequence {
              tunnel: [w313] -> w310
              tunnel: [w319] -> w311
              tunnel: w310 -> [w319]
              frame #0 {
                n159 = global read "VAR总磷氨氮全局变量.vi" "状态告警区"() -> (w316:T3)
                n160 = Unbundle By Name(w316) -> ("工作状态"=w317:T7)
                n161 = Equal To 0?(x=w317) -> (x = 0?=w312:bool)
                n162 = Select(t=T4."延时", s=w312, f=T4."总磷测量中") -> (s? t:f=w313:T4)
              }
              frame #1 {
                n163 = Wait (ms)(milliseconds to wait=u32 5000 ("等待时间（毫秒）")) -> ()  [unwired: 1 out]
              }
            }
          }
          frame "延时" {
            n164 = local read "设置值"() -> (w325:dbl)
            n165 = Increment(x=w326) -> (x+1=w322:u32)
            n166 = Greater Or Equal?(x=w322, y=w325) -> (x >= y?=w324:bool)
            n167 = Select(t=T4."待机", s=w324, f=T4."延时") -> (s? t:f=w323:T4)
          }
        }
      }
    }
  }
  n168 = while {
    tunnel: w34 -> [w333]
    tunnel: w14 -> [w332]
    tunnel: w13 -> [w331]
    tunnel: w12 -> [w330]
    tunnel: w11 -> [w329]
    tunnel: w10 -> [w328]
    tunnel: w9 -> [w327]
    tunnel: w7 -> [_]
    stop <- FALSE stop-if-true
    n169 = event shown="[1] \"手动启动\": 值改变" {
      selector: _ -> [_ _ _ _ _ _ _ _ _ _ _ _ _ _ _]
      dyn-events: _ -> [_ _ _ _ _ _ _ _ _ _ _ _ _ _ _]
      timeout: _ -> [_ _ _ _ _ _ _ _ _ _ _ _ _ _ _]
      tunnel: w333 -> [_ w337 _ w348 w350 _ _ _ _ _ _ _ _ _ _]
      tunnel: w332 -> [_ _ _ _ _ _ _ _ _ w403 _ w423 w432 _ _]
      tunnel: w331 -> [_ _ _ _ _ _ _ _ _ w401 _ w421 w434 w442 w449]
      tunnel: w330 -> [_ _ _ _ _ _ _ _ _ w402 _ w422 w433 _ _]
      tunnel: w329 -> [_ _ _ _ _ _ _ _ _ w397 _ _ _ _ _]
      tunnel: w328 -> [_ _ _ _ _ _ _ _ _ _ _ w417 _ _ _]
      tunnel: w327 -> [_ _ _ _ _ _ _ _ _ _ _ _ _ w440 _]
      event Timeout {
        n170 = event-data() -> ()  [unwired: 1 in, 3 out]
      }
      event "手动启动": Value Change {
        n171 = event-data() -> ()  [unwired: 1 in, 6 out]
        n172 = call "总磷氨氮启动参数对话框.vi"() -> ("确认"=w335:bool, "元素"=w336:cluster{"命令":string, "data":variant})  [unwired: 10 in]
        n173 = case shown="真" w335 {
          tunnel: w337 -> [_ w339]
          tunnel: w336 -> [_ w338]
          frame False {
          }
          frame True {
            n174 = Enqueue Element(queue=w339, element=w338) -> ()  [unwired: 2 in, 3 out]
          }
        }
      }
      event "定时启动": Mouse Down {
        n175 = event-data() -> ()  [unwired: 1 in, 6 out]
        n176 = call "定时启动对话框.vi"() -> ("设置值"=→"设置值":dbl, "确定输出"=→"定时启动":bool)  [unwired: 10 in]
      }
      event "单步测试": Value Change {
        w343 = u16 1 items=["总磷"=1, "氨氮"=3] ("站号")
        n177 = event-data() -> ()  [unwired: 1 in, 6 out]
        n178 = Bundle("站号"=w343, "总磷氨氮调试"="总磷氨氮调试") -> (w342:cluster{"站号":u16, "总磷氨氮调试":u16[]})  [unwired: 1 in]
        n179 = Bundle By Name(cluster=cluster{"命令":string, "data":variant} {"命令"="", "data"=variant} ("元素"), "命令"="debug", "data"=w342) -> (w345:cluster{"命令":string, "data":variant})
        n180 = Enqueue Element(queue=w348, element=w345) -> ()  [unwired: 2 in, 3 out]
      }
      event "停止": Value Change {
        n181 = event-data() -> ()  [unwired: 1 in, 6 out]
        n182 = Enqueue Element(queue=w350, element=cluster{"命令":string, "data":variant} {"命令"="启动", "data"=variant(cluster{"站号":u16, "控制命令输出":u16[]} {"站号"=1, "控制命令输出"=[2816]})} ("元素")) -> ()  [unwired: 2 in, 3 out]
      }
      event "调试": Value Change {
        n183 = event-data() -> ()  [unwired: 1 in, 6 out]
        n184 = property on="窗格" class="Pane"("Origin"=T5 {"Horizontal"=0, "Vertical"=432} ("原点")) -> ()  [unwired: 2 in, 2 out]
      }
      event "返回": Value Change {
        n185 = event-data() -> ()  [unwired: 1 in, 6 out]
        n186 = property on="窗格" class="Pane"("Origin"=T5 {"Horizontal"=0, "Vertical"=0} ("原点")) -> ()  [unwired: 2 in, 2 out]
      }
      event "标液浓度1", "测量吸光度1", "测量吸光度2", "标液浓度2", "测量吸光度3", "标液浓度3", "测量吸光度4", "标液浓度4", "测量吸光度5", "标液浓度5", "样品1启用", "样品3启用", "样品4启用", "样品5启用", "样品2启用", "模型", "method", "样品1 F0", "样品1 F1", "样品2 F1", "样品2 F0", "样品3 F1", "样品4 F0", "样品4 F1", "样品5 F1", "样品5 F0", "精度": Value Change {
        n187 = event-data() -> ()  [unwired: 1 in, 6 out]
        n188 = formula code="E=log(F0/F1);"("F0"="样品1 F0", "F1"="样品1 F1") -> ("E"=w374:dbl)
        "测量吸光度1" <- w374
        n189 = formula code="E=log(F0/F1);"("F0"="样品2 F0", "F1"="样品2 F1") -> ("E"=w371:dbl)
        "测量吸光度2" <- w371
        n190 = formula code="E=log(F0/F1);"("F0"="样品3 F0", "F1"="样品3 F1") -> ("E"=w368:dbl)
        "测量吸光度3" <- w368
        n191 = formula code="E=log(F0/F1);"("F0"="样品4 F0", "F1"="样品4 F1") -> ("E"=w365:dbl)
        "测量吸光度4" <- w365
        n192 = formula code="E=log(F0/F1);"("F0"="样品5 F0", "F1"="样品5 F1") -> ("E"=w362:dbl)
        "测量吸光度5" <- w362
        n193 = Replace Array Subset(array=dbl[] [0.0, 0.0, 0.0, 0.0, 0.0] ("数组"), new element #1="标液浓度1", new element #2="标液浓度2", new element #3="标液浓度3", new element #4="标液浓度4", new element #5="标液浓度5") -> (w359:dbl[])  [unwired: 5 in]
        n194 = Replace Array Subset(array=dbl[] [0.0, 0.0, 0.0, 0.0, 0.0] ("数组"), new element #1=w374, new element #2=w371, new element #3=w368, new element #4=w365, new element #5=w362) -> (w358:dbl[])  [unwired: 5 in]
        n195 = Replace Array Subset(array=bool[] [FALSE, FALSE, FALSE, FALSE, FALSE] ("数组"), new element #1="样品1启用", new element #2="样品2启用", new element #3="样品3启用", new element #4="样品4启用", new element #5="样品5启用") -> (w357:bool[])  [unwired: 5 in]
        n196 = call "线性公式.vi"("精度"="精度", "模型"="模型", "method"="method", "启用"=w357, "监测浓度"=w358, "标液浓度"=w359) -> ("XY图"=→"XY图":cluster{"X Values":dbl[], "Y Values":dbl[]}[], "r^2"=→"r^2":dbl, "拟合方程"=→"拟合公式":string)  [unwired: 3 in]
      }
      event "标液浓度1", "标液浓度2", "标液浓度3", "标液浓度4", "标液浓度5", "样品1 F0", "样品1 F1", "样品2 F1", "样品2 F0", "样品3 F1", "样品3 F0", "样品4 F0", "样品4 F1", "样品5 F0", "样品5 F1", "精度", "公式.X^2", "公式.X", "公式.b", "量程切换阈值.阈值", "量程切换阈值.标液浓度", "备用系数.量程上限", "备用系数.量程下限", "备用系数.检出限", "备用系数.精度": Mouse Down {
        n197 = event-data() -> ("CtlRef"=w393:refnum<vi>)  [unwired: 1 in, 5 out]
        n198 = property class="DigNum (严格)"(reference=w393) -> (reference out=w391:refnum<vi>, "Value"=w392:dbl)  [unwired: 1 in, 1 out]
        n199 = call "数字键盘.vi"("OldNumber"=w392) -> ("NewNumber"=w390:sgl)
        n200 = property class="DigNum (严格)"(reference=w391, "Val(Sgnl)"=w390) -> ()  [unwired: 1 in, 2 out]
      }
      event "读公式": Value Change {
        n201 = event-data() -> ()  [unwired: 1 in, 6 out]
        n202 = property class="Enum (严格)"(reference=w401) -> ("Value"=w400:enum16{"氨氮", "总磷"})  [unwired: 1 in, 2 out]
        n203 = property class="Enum (严格)"(reference=w402) -> ("Value"=w399:enum16{"水样测量", "空白核查", "标样核查", "盲样测试", "加标回收"})  [unwired: 1 in, 2 out]
        n204 = property class="Enum (严格)"(reference=w403) -> ("Value"=w398:enum16{"低量程", "高量程"})  [unwired: 1 in, 2 out]
        n205 = call "总磷氨氮公式读取.vi"("量程"=w398, "测量模式"=w399, "测量参数"=w400) -> ("error out"=w395:errorcluster, "公式"=w396:cluster{"X^2":dbl, "X":dbl, "b":dbl})  [unwired: 7 in]
        n206 = property class="Clust (严格)"(reference=w397, "Value"=w396) -> ()  [unwired: 1 in, 2 out]
        n207 = case shown="错误" w395 {
          tunnel: ["读取成功" ("消息") "读取失败" ("消息")] -> w394
          frame No Error {
          }
          frame Error {
          }
        }
        n208 = One Button Dialog(message=w394) -> ()  [unwired: 1 in, 1 out]
      }
      event "写公式": Value Change {
        n209 = event-data() -> ()  [unwired: 1 in, 6 out]
        n210 = call "总磷氨氮公式写入.vi"("公式"="公式", "量程"="量程下拉列表", "测量模式"="测量模式下拉列表", "测量参数"="参数下拉列表") -> ("error out"=w406:errorcluster)  [unwired: 7 in]
        n211 = case shown="无错误" w406 {
          tunnel: ["写入成功" ("消息") "写入失败" ("消息")] -> w407
          frame No Error {
          }
          frame Error {
          }
        }
        n212 = One Button Dialog(message=w407) -> ()  [unwired: 1 in, 1 out]
      }
      event "量程切换阈值读取": Value Change {
        n213 = event-data() -> ()  [unwired: 1 in, 6 out]
        n214 = property class="Enum (严格)"(reference=w421) -> ("Value"=w420:enum16{"氨氮", "总磷"})  [unwired: 1 in, 2 out]
        n215 = property class="Enum (严格)"(reference=w422) -> ("Value"=w419:enum16{"水样测量", "空白核查", "标样核查", "盲样测试", "加标回收"})  [unwired: 1 in, 2 out]
        n216 = property class="Enum (严格)"(reference=w423) -> ("Value"=w418:enum16{"低量程", "高量程"})  [unwired: 1 in, 2 out]
        n217 = call "总磷氨氮量程读取.vi"("量程"=w418, "测量模式"=w419, "测量参数"=w420) -> ("error out"=w414:errorcluster, "量程切换阈值"=w416:cluster{"阈值":dbl, "标液浓度":dbl})  [unwired: 7 in]
        n218 = property class="Clust (严格)"(reference=w417, "Value"=w416) -> ()  [unwired: 1 in, 2 out]
        n219 = case shown="错误" w414 {
          tunnel: ["读取成功" ("消息") "读取失败" ("消息")] -> w415
          frame No Error {
          }
          frame Error {
          }
        }
        n220 = One Button Dialog(message=w415) -> ()  [unwired: 1 in, 1 out]
      }
      event "量程切换阈值写入": Value Change {
        n221 = event-data() -> ()  [unwired: 1 in, 6 out]
        n222 = property class="Enum (严格)"(reference=w434) -> ("Value"=w431:enum16{"氨氮", "总磷"})  [unwired: 1 in, 2 out]
        n223 = property class="Enum (严格)"(reference=w433) -> ("Value"=w430:enum16{"水样测量", "空白核查", "标样核查", "盲样测试", "加标回收"})  [unwired: 1 in, 2 out]
        n224 = property class="Enum (严格)"(reference=w432) -> ("Value"=w429:enum16{"低量程", "高量程"})  [unwired: 1 in, 2 out]
        n225 = call "总磷氨氮量程写入.vi"("量程切换阈值"="量程切换阈值", "量程"=w429, "测量模式"=w430, "测量参数"=w431) -> ("error out"=w426:errorcluster)  [unwired: 7 in]
        n226 = case shown="无错误" w426 {
          tunnel: ["写入成功" ("消息") "写入失败" ("消息")] -> w427
          frame No Error {
          }
          frame Error {
          }
        }
        n227 = One Button Dialog(message=w427) -> ()  [unwired: 1 in, 1 out]
      }
      event "备用系数读取": Value Change {
        n228 = event-data() -> ()  [unwired: 1 in, 6 out]
        n229 = property class="Enum (严格)"(reference=w442) -> ("Value"=w441:enum16{"氨氮", "总磷"})  [unwired: 1 in, 2 out]
        n230 = call "总磷氨氮备用系数读取.vi"("测量参数"=w441) -> ("error out"=w437:errorcluster, "备用系数"=w439:T1)  [unwired: 9 in]
        n231 = property class="Clust (严格)"(reference=w440, "Value"=w439) -> ()  [unwired: 1 in, 2 out]
        n232 = case shown="错误" w437 {
          tunnel: ["读取成功" ("消息") "读取失败" ("消息")] -> w438
          frame No Error {
          }
          frame Error {
          }
        }
        n233 = One Button Dialog(message=w438) -> ()  [unwired: 1 in, 1 out]
      }
      event "备用系数写入": Value Change {
        n234 = event-data() -> ()  [unwired: 1 in, 6 out]
        n235 = property class="Enum (严格)"(reference=w449) -> ("Value"=w448:enum16{"氨氮", "总磷"})  [unwired: 1 in, 2 out]
        n236 = call "总磷氨氮备用系数写入.vi"("备用系数"="备用系数", "测量参数"=w448) -> ("error out"=w445:errorcluster)  [unwired: 9 in]
        n237 = case shown="无错误" w445 {
          tunnel: ["写入成功" ("消息") "写入失败" ("消息")] -> w446
          frame No Error {
          }
          frame Error {
          }
        }
        n238 = One Button Dialog(message=w446) -> ()  [unwired: 1 in, 1 out]
      }
    }
  }
  n239 = while {
    tunnel: w34 -> [w467]
    tunnel: w35 -> [_]
    shift-right: [w460] -> _
    shift-left: enum16{"氨氮", "总磷"}."氨氮" ("枚举") -> [w461]
    stop <- FALSE stop-if-true
    w462 = u16 1 items=["总磷"=1, "氨氮"=3] ("站号")
    # "试剂填充 172 \n管路清洗108\n氨氮92\n总磷131\n总磷海水147\n总氮76\n总氮海水92"
    n240 = Wait (ms)(milliseconds to wait=u32 1000 ("等待时间（毫秒）")) -> ()  [unwired: 1 out]
    n241 = Bundle By Name(cluster=cluster{"命令":string, "data":variant} {"命令"="", "data"=variant} ("元素"), "命令"="读状态告警区", "data"=w462) -> (w469:cluster{"命令":string, "data":variant})
    n242 = global read "VAR总磷氨氮全局变量.vi" "状态告警区"() -> (w458:T3)
    n243 = Bundle By Name(cluster=cluster{"命令":string, "data":variant} {"命令"="", "data"=variant} ("元素"), "命令"="读测量数据区", "data"=w462) -> (w465:cluster{"命令":string, "data":variant})
    n244 = Unbundle By Name(w458) -> ("系统时间"=w457:timestamp)
    n245 = Enqueue Element(queue=w467, element=w469) -> (queue out=w463:refnum<queue>)  [unwired: 2 in, 2 out]
    n246 = Enqueue Element(queue=w463, element=w465) -> (queue out=w459:refnum<queue>)  [unwired: 2 in, 2 out]
    n247 = Get Date/Time In Seconds() -> (seconds since 1Jan1904=w456:timestamp)
    n248 = Subtract(x=w457, y=w456) -> (x-y=w455:dbl)
    n249 = Absolute Value(x=w455) -> (abs(x)=w454:dbl)
    n250 = Greater Or Equal?(x=w454, y=120.0) -> (x >= y?=w452:bool)
    n251 = case shown="真" w452 {
      tunnel: w459 -> [_ w473]
      frame False {
      }
      frame True {
        n252 = call "总磷氨氮启动命令.vi"("参数"=T17 {"站号"=1, "量程切换"=enum."AUTO", "控制命令"=enum."校时", "模式设置"=enum."待机", "测量间隔"=0}) -> ("启动命令"=w474:cluster{"命令":string, "data":variant})  [unwired: 10 in]
        n253 = Enqueue Element(queue=w473, element=w474) -> ()  [unwired: 2 in, 3 out]
      }
    }
    n254 = Increment(x=w461) -> (x+1=w460:enum16{"氨氮", "总磷"})
  }
  n255 = Open VI Reference(type specifier VI Refnum (for type only)=refnum<vi> refnum, vi path=w16, options=128 ("选项")) -> (vi reference=w18:refnum<vi>, error out=w20:errorcluster)  [unwired: 3 in]
  n256 = Close Reference(reference=w24, error in (no error)=w25) -> ()  [unwired: 1 out]
  n257 = call-by-ref "?"(reference=w18, error in=w20) -> (reference out=w22:refnum<vi>, error out=w21:errorcluster)  [unwired: 12 in]
  n258 = Close Reference(reference=w22, error in (no error)=w21) -> ()  [unwired: 1 out]
  n259 = node-c288(w4) -> ()  [unwired: 1 out]
